vi "Error (IDL).vi"(7 "Previous step":T1, 8 "Error In":errorcluster, 11 "Queue In":refnum<queue>) -> (0 "Error Out":errorcluster, 2 "Error data":variant, 3 "Queue Out":refnum<queue>)   [LabVIEW 2018, in "Tracker.lvlib"]
uses:
  Tracker.lvlib
  Controls/CTL_Control_States.ctl
  Common_Resources.lvlib
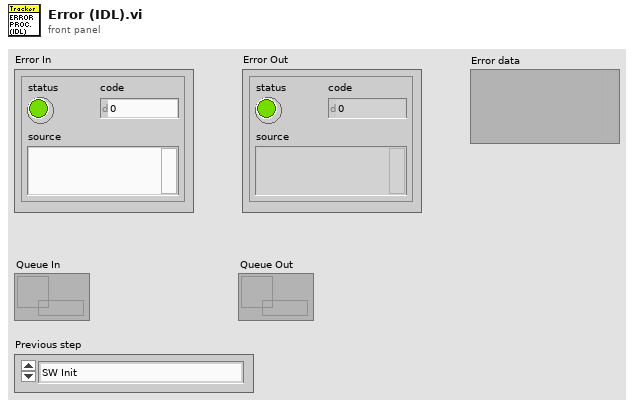
[diagram p1: front panel]
types:
  T1 = typedef "Common_Resources.lvlib/CTL_Control_States.ctl" = enum16{"SW Init", "HW Init", "Close App", "Update port info (Init OK)", "Unlock UI (init OK)", "Save HW Settings", "Re-check HW (init failed)", "Configure port(s)", "Switch to Offline mode", "Switch to Online mode", "Zones layout update", "Set I/O config (silent)", "Set I/O config", "Play Start", "Play Stop", "Upd. FPS", "Upd. trace length", "Cage and recording settings", "Update filter", "Timings calibration start", "Timings calibration finish", "Dispension calibration", "Save all settings to custom location", "Save all settings", "Start Recording", "Stop Recording", "Recording post-processing", "Timeline update", "Overlay tracks update", "Load custom settings", "Load recorded data", "Save density map(s)", "Process loaded settings", "Prepare loaded data playback", "Add Reward condition", "Modify Reward condition", "Delete Reward condition", "Check Reward condition(s)", "Location map update", "Speed map update", "Start over", "Default (test)", "IDL Error", "Recalculate track with new settings"}
  T2 = cluster{"Previous step":T1, "error IO":errorcluster}
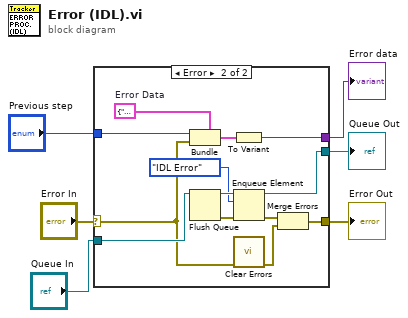
[diagram p0: block diagram]
diagram:
  n1 = case shown="Error" "Error In" {
    selector: "Error In" -> [w8 w12]
    tunnel: [w8 w15] -> w5
    tunnel: "Queue In" -> [w7 w21]
    tunnel: [w7 w18] -> w3
    tunnel: "Previous step" -> [_ w11]
    tunnel: [_ w13] -> w1
    frame No Error {
    }
    frame Error {
      w9 = T2 {"Previous step"=enum."SW Init", "error IO"={"status"=FALSE, "code"=0, "source"=""}}  # Error Data
      n2 = Bundle(cluster=w9, "Previous step"=w11, "error IO"=w12) -> (w10:T2)
      n3 = Flush Queue(queue=w21) -> (queue out=w20:refnum<queue>, error out=w16:errorcluster)  [unwired: 1 in, 1 out]
      n4 = To Variant(anything=w10) -> (Variant=w13:variant)
      n5 = Enqueue Element(queue=w20, element=CTL_Control_States."IDL Error", error in (no error)=w16) -> (queue out=w18:refnum<queue>, error out=w14:errorcluster)  [unwired: 1 in, 1 out]
      n6 = call <vilib>:"Clear Errors.vi"("error in (no error)"=w12) -> ("error out"=w17:errorcluster)  [unwired: 5 in, 1 out]
      n7 = Merge Errors(w14, w17) -> (w15:errorcluster)
    }
  }
  "Error Out" <- w5
  "Queue Out" <- w3
  "Error data" <- w1
